vi "02 Occurences and more.vi"() -> ()   [LabVIEW 2019]
uses:
  examples/Synchronization/Occurrence/support/Global - Occurrence Loop Stop.vi
panel:
  out "Total Occurrences Fired":i32
  out "Current Loop 1 Iteration":i32
  in  "Stop":bool
  # "Hit the Run arrow and see the Gauge change to the value of the Slide\n\nHit Continuous Run and watch the Gauge change as you vary the Slide"
  # "Hit Cmd E to see the diagram (code)"
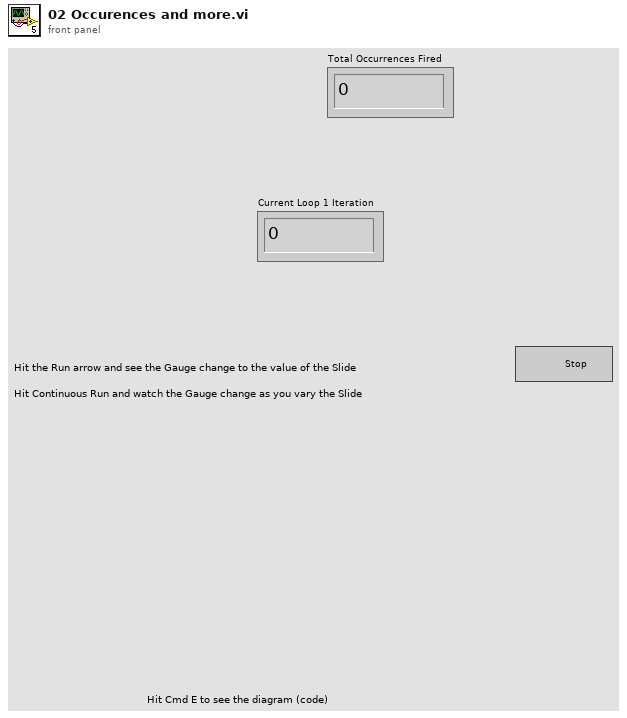
[diagram p1: front panel]
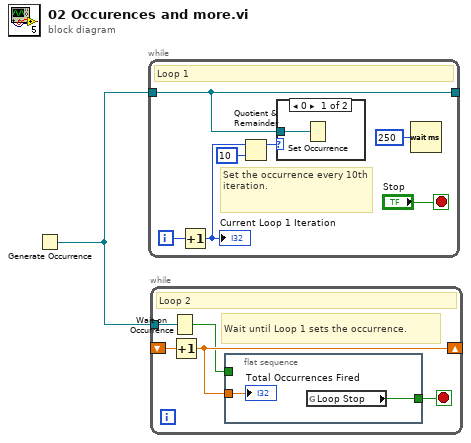
[diagram p0: block diagram]
diagram:
  n1 = Generate Occurrence() -> (w1:refnum<k4>)
  n2 = while {
    tunnel: w1 -> [w4]
    tunnel: [w4] -> _
    i -> [w8]
    stop <- "Stop" stop-if-true
    # "Set the occurrence every 10th iteration."
    # "Loop 1"
    n3 = Increment(x=w8) -> (x+1=w7:i32)
    "Current Loop 1 Iteration" <- w7
    n4 = Quotient & Remainder(x=w7, y=10) -> (x-y*floor(x/y)=w5:i32)  [unwired: 1 out]
    n5 = case shown="0" w5 {
      tunnel: w4 -> [w9 _]
      frame 0 {
        n6 = Set Occurrence(w9) -> ()
      }
      frame Default {
      }
    }
    n7 = Wait (ms)(milliseconds to wait=u32 250) -> ()  [unwired: 1 out]
  }
  n8 = while {
    tunnel: w1 -> [w14]
    shift-right: [w12] -> _
    shift-left: _ -> [w13]
    stop <- w11 stop-if-true
    # "Wait until Loop 1 sets the occurrence."
    # "Loop 2"
    n9 = Wait on Occurrence(2:w14) -> (0:w10:bool)  [unwired: 2 in]
    n10 = Increment(x=w13) -> (x+1=w12:dbl)
    n11 = flat-sequence {
      tunnel: w12 -> [w16]
      tunnel: [w15] -> w11
      tunnel: w10 -> [_]
      frame #0 {
        n12 = global read "Global - Occurrence Loop Stop.vi" "Loop Stop"() -> (w15:bool)
        "Total Occurrences Fired" <- w16
      }
    }
  }
